vi "VCS Analog Input Configuration.vi"(0 "axis in":cluster{"keyHandle":u32, "nodeId":u16}={"keyHandle"=0, "nodeId"=1}, 7 "configuration":T1={"analogInputNumber"=1, "configuration"=15, "executionMask"=0} {"executionMask" items=["disabled", "enabled"]; "configuration" items=["current setpoint"=0, "velocity setpoint"=1, "position setpoint"=2, "general purpose A"=15, "general purpose B"=14, "general purpose C"=13, "general purpose D"=12, "general purpose E"=11, "general purpose F"=10, "general purpose G"=9, "general purpose H"=8]}, 11 "error in (no error)":errorcluster) -> (4 "axis out":cluster{"keyHandle":u32, "nodeId":u16}={"keyHandle"=0, "nodeId"=1}, 15 "error out":errorcluster)   [LabVIEW 2019, in "maxonEPOS.lvlib"]
doc: "<B>VCS_AnalogInputConfiguration</B> sets parameter for one analog input."
uses:
  Examples/maxonEPOS.lvlib
  Resources/EposCmd.dll
  Resources/EposCmd64.dll
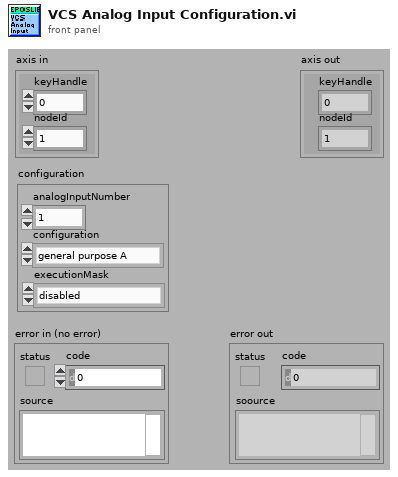
[diagram p1: front panel]
types:
  T1 = cluster{"analogInputNumber":u16, "configuration":u16, "executionMask":i32}
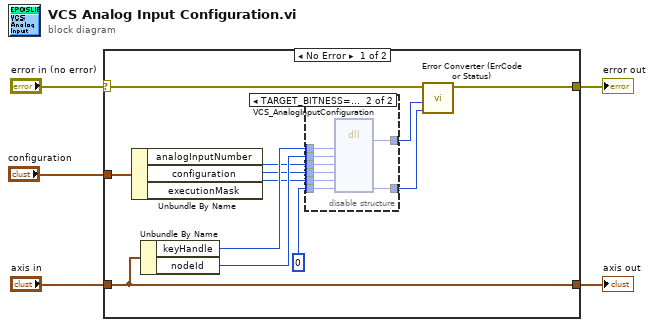
[diagram p0: block diagram]
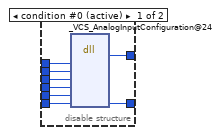
[diagram p2: hidden frame]
diagram:
  n1 = case shown="No Error" "error in (no error)" {
    selector: "error in (no error)" -> [w15 w34]
    tunnel: "axis in" -> [w17 w35]
    tunnel: [w17 w35] -> w4
    tunnel: [w16 w34] -> w3
    tunnel: "configuration" -> [w9 _]
    frame No Error {
      n2 = Unbundle By Name(w9) -> ("analogInputNumber"=w8:u16, "configuration"=w7:u16, "executionMask"=w6:i32)
      n3 = Unbundle By Name(w17) -> ("keyHandle"=w12:u32, "nodeId"=w13:u16)
      n4 = disable-structure shown="TARGET_BITNESS==64" {
        disable-tunnel: u32 0 ("pErrorCode") -> [w25 w33]
        disable-tunnel: w13 -> [w24 w32]
        disable-tunnel: w12 -> [w23 w31]
        disable-tunnel: [w22 w30] -> w11
        disable-tunnel: [w21 w29] -> w10
        disable-tunnel: w8 -> [w20 w28]
        disable-tunnel: w7 -> [w19 w27]
        disable-tunnel: w6 -> [w18 w26]
        frame condition #0 (active) {
          n5 = dll-call lib="C:/workspace/project/scancon/sw/SSI_Tool/InstrumentsInterfaces/Motordriver/maxon EPOS/Resources/EposCmd.*" fn="_VCS_AnalogInputConfiguration@24"("KeyHandle"=w23, "NodeId"=w24, "AnlogInputNb"=w20, "Configuration"=w19, "ExecutionMask"=w18, "pErrorCode"=w25) -> (w22:i32, "pErrorCode"=w21:u32)  [unwired: 8 in, 2 out]
        }
        frame condition #1 {
          n6 = dll-call lib="C:/Sources/LabView/maxon EPOS/Resources/EposCmd64.*" fn="VCS_AnalogInputConfiguration" ("EposCmd.dll:_VCS_AnalogInputConfiguration@24")("KeyHandle"=w31, "NodeId"=w32, "AnlogInputNb"=w28, "Configuration"=w27, "ExecutionMask"=w26, "pErrorCode"=w33) -> ("Rückgabetyp"=w30:i32, "pErrorCode"=w29:u32)  [unwired: 8 in, 2 out]
        }
      }
      n7 = call "Error Converter (ErrCode or Status).vi"("error code"=w10, "return type"=w11, "error in (no error)"=w15) -> ("error out"=w16:errorcluster)  [unwired: 7 in]
    }
    frame Error {
    }
  }
  "error out" <- w3
  "axis out" <- w4
